vi "Text Style Init.vi"(10 "Text Style Value":T1={"Font"="", "Size"=0.0, "Justification"=1, "TextColor"=0, "BGColor"=0, "Bold"=FALSE}, 11 "Text Style Ctrl":refnum<vi>) -> ()   [LabVIEW 2015, in "UIStep.lvclass"]
uses:
  UIStep.lvclass
  <vilib>/registry/registry.llb/Registry RtKey.ctl
  <vilib>/registry/registry.llb/Registry SAM.ctl
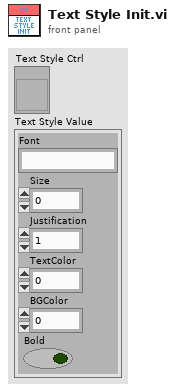
[diagram p1: front panel]
types:
  T1 = cluster{"Font":string, "Size":dbl, "Justification":u16, "TextColor":u32, "BGColor":u32, "Bold":bool}
  T2 = typedef "Registry SAM.ctl" = enum32{"KEY_QUERY_VALUE", "KEY_SET_VALUE", "KEY_CREATE_SUB_KEY", "KEY_ENUMERATE_SUB_KEYS", "KEY_NOTIFY", "KEY_CREATE_LINK", "KEY_READ", "KEY_WRITE", "KEY_ALL_ACCESS", "KEY_READ | KEY_WRITE"}
  T3 = typedef "Registry RtKey.ctl" = enum32{"HKEY_CLASSES_ROOT", "HKEY_CURRENT_USER", "HKEY_LOCAL_MACHINE", "HKEY_USERS", "HKEY_PERFORMANCE_DATA", "HKEY_CURRENT_CONFIG", "HKEY_DYN_DATA"}
  T4 = typedef "Registry refnum.ctl" = refnum<k1>
  T5 = cluster{"numValues":i32, "maxValueNameLen":i32, "maxValueDataLen":i32}
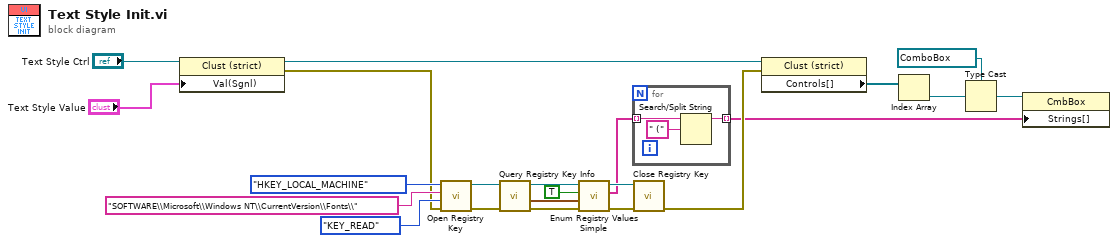
[diagram p0: block diagram]
diagram:
  n1 = property class="Clust (strict)"(reference="Text Style Ctrl", "Val(Sgnl)"="Text Style Value") -> (reference out=w20:refnum<vi>, error out=w3:errorcluster)  [unwired: 1 in]
  n2 = call <vilib>:"Open Registry Key.vi"("error in (no error)"=w3, "security access mask (KEY_READ | KEY_WRITE)"=Registry_SAM."KEY_READ", "subkey"="SOFTWARE\\Microsoft\\Windows NT\\CurrentVersion\\Fonts\\", "root key (HKEY_LOCAL_MACHINE)"=Registry_RtKey."HKEY_LOCAL_MACHINE") -> ("error out"=w13:errorcluster, "refnum out"=w14:T4)  [unwired: 6 in]
  n3 = call <vilib>:"Query Registry Key Info.vi"("error in (no error)"=w13, "refnum"=w14) -> ("error out"=w10:errorcluster, "value info"=w7:T5, "refnum out"=w11:T4)  [unwired: 5 in, 2 out]
  n4 = call <vilib>:"Enum Registry Values Simple.vi"("error in (no error)"=w10, "value info"=w7, "retrieve data? (F)"=TRUE, "refnum"=w11) -> ("error out"=w9:errorcluster, "values"=w5:string[], "refnum out"=w8:T4)  [unwired: 2 in, 3 out]
  n5 = for {
    tunnel: w5 -> [w25] mode=indexing
    tunnel: [w23] -> w1 mode=indexing
    n6 = Search/Split String(string=w25, search string/char (-)=" (") -> (substring before match=w23:string)  [unwired: 1 in, 2 out]
  }
  n7 = call <vilib>:"Close Registry Key.vi"("error in (no error)"=w9, "refnum"=w8) -> ("error out"=w2:errorcluster)  [unwired: 5 in]
  n8 = property class="Clust (strict)"(reference=w20, error in=w2) -> ("Controls[]"=w19:refnum<vi>[])  [unwired: 2 out]
  n9 = Index Array(array=w19) -> (element=w18:refnum<vi>)  [unwired: 1 in]
  n10 = Type Cast(type=refnum<vi> refnum ("element"), x=w18) -> (*(type *) &x=w16:refnum<vi>)
  n11 = property class="CmbBox"(reference=w16, "Strings[]"=w1) -> ()  [unwired: 1 in, 2 out]
